vi "Abort.vi"(8 "error in (no error)":errorcluster, 11 "LUnit Test Case in":refnum<class "LUnit Test Case.lvclass">) -> (0 "error out":errorcluster)   [LabVIEW 2020, in "LUnit Test Case.lvclass"]
uses:
  LUnit Test Case.lvclass
  LUnit Test Case.lvclass/LUnit Test Case.ctl
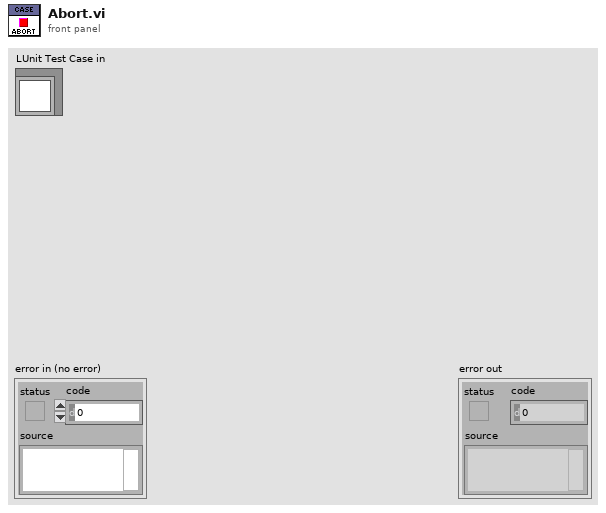
[diagram p1: front panel]
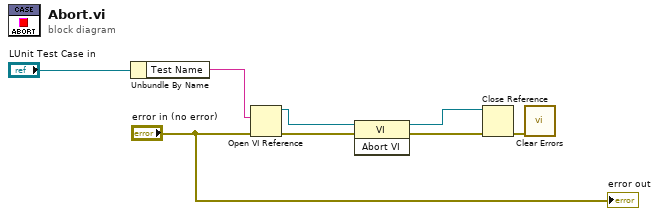
[diagram p0: block diagram]
diagram:
  n1 = Unbundle By Name("LUnit Test Case in") -> ("Test Name"=w5:string)
  n2 = Open VI Reference(vi path=w5, error in (no error)="error in (no error)") -> (vi reference=w4:refnum<vi>, error out=w6:errorcluster)  [unwired: 4 in]
  n3 = invoke class="VI" method="Abort VI"(reference=w4, error in=w6) -> (reference out=w2:refnum<vi>, error out=w7:errorcluster)  [unwired: 1 in, 1 out]
  n4 = Close Reference(reference=w2, error in (no error)=w7) -> (error out=w3:errorcluster)
  n5 = call <vilib>:"Clear Errors.vi"("error in (no error)"=w3) -> ()  [unwired: 5 in, 2 out]
  "error out" <- "error in (no error)"
